vi "Find task.vi"(7 "Function":string="SA path selector", 8 "error in (no error)":errorcluster, 11 "NI USB-6501 in":refnum<class "NI USB-6501.lvclass">) -> (0 "error out":errorcluster, 2 "Task":refnum<k21>, 3 "NI USB-6501 out":refnum<class "NI USB-6501.lvclass">)   [LabVIEW 2020, in "NI USB-6501.lvclass"]
uses:
  NI USB-6501.lvclass
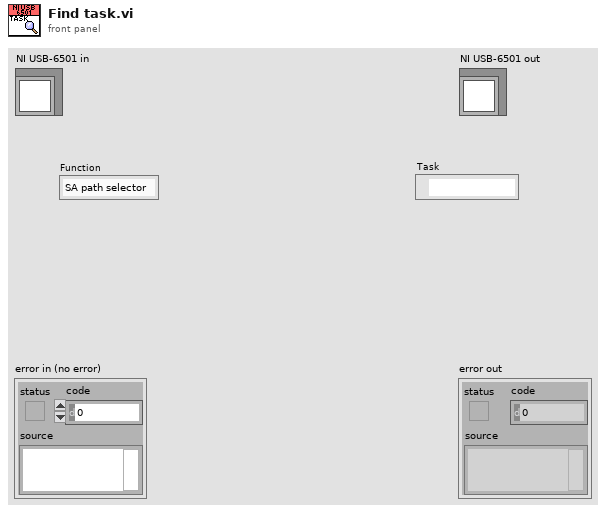
[diagram p1: front panel]
types:
  T1 = typedef "NI USB-6501.lvclass/Channel.ctl" = cluster{"Channel":tag, "Task":refnum<k21>, "Function":string, "Low":string, "High":string, "Direction":enum16{"Input", "Output"}}
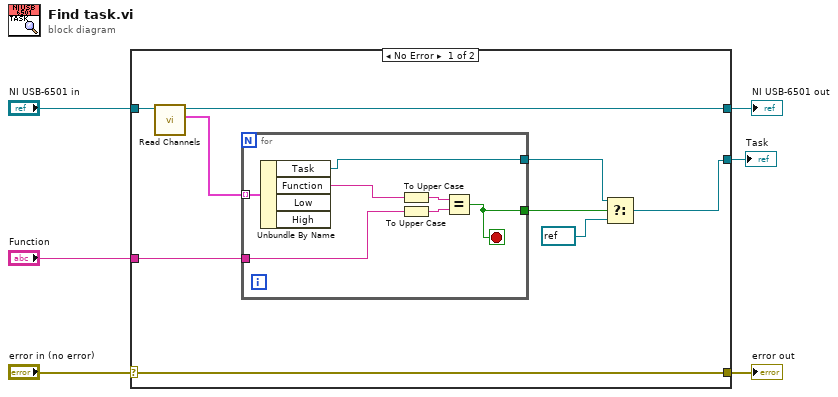
[diagram p0: block diagram]
diagram:
  n1 = case shown="No Error" "error in (no error)" {
    selector: "error in (no error)" -> [w15 w24]
    tunnel: [w15 w24] -> w5
    tunnel: [w12 w23] -> w3
    tunnel: "NI USB-6501 in" -> [w13 w23]
    tunnel: "Function" -> [w11 _]
    tunnel: [w8 _] -> w1
    frame No Error {
      n2 = call-dynamic "Read Channels.vi"("NI USB-6501 in"=w13) -> ("Channels"=w14:T1[], "NI USB-6501 out"=w12:refnum<class "NI USB-6501.lvclass">)  [unwired: 9 in]
      n3 = for {
        tunnel: w14 -> [w22] mode=indexing
        tunnel: [w18] -> w10
        tunnel: w11 -> [w17]
        tunnel: [w16] -> w9
        stop <- w18 stop-if-true
        n4 = Unbundle By Name(w22) -> ("Task"=w16:refnum<k21>, "Function"=w21:string)  [unwired: 2 out]
        n5 = To Upper Case(1:w21) -> (0:w20:string)
        n6 = To Upper Case(1:w17) -> (0:w19:string)
        n7 = Equal?(x=w20, y=w19) -> (x = y?=w18:bool)
      }
      n8 = Select(t=w9, s=w10, f=refnum<k21> refnum) -> (s? t:f=w8:refnum<k21>)
    }
    frame Error {
    }
  }
  "error out" <- w5
  "NI USB-6501 out" <- w3
  "Task" <- w1
